vi "Calibrate Sensor Angle.vi"() -> ()   [LabVIEW 2014]
uses:
  <vilib>/Utility/AngleManip/Degrees to Radians (Scalar DBL).vi
  <vilib>/robotics/Starter Kit/2.0/9632 Host Interface/NI_Robotics_Starter Kit Host_9632_2.0.lvclass
  <vilib>/Utility/AngleManip/NI_AngleManipulation.lvlib
  <vilib>/robotics/Starter Kit/Host Interface/NI_Robotics_Starter Kit Host.lvclass
panel:
  in  "sensor motor angle":dbl(slide) caption="Sensor Motor Angle (degrees)" scale=90.0..-90.0
  in  "zero":bool
  in  "stop":bool
  # "Adjust the slider until the sensor is facing directly forward on the robot, then press Zero Angle to calibrate the sensor orientation."
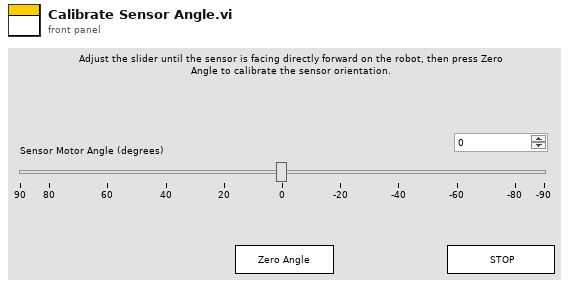
[diagram p1: front panel]
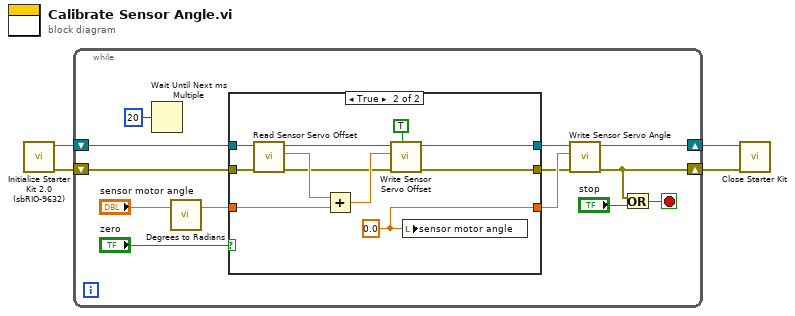
[diagram p0: block diagram]
diagram:
  n1 = call <vilib>:"Initialize Starter Kit 2.0 (sbRIO-9632).vi"() -> ("error out"=w3:errorcluster, "FPGA starter kit host 2.0 out"=w4:refnum<class "NI_Robotics_Starter Kit Host_9632_2.0.lvclass">)  [unwired: 10 in]
  n2 = while {
    shift-right: [w6] -> w2
    shift-left: w4 -> [w13]
    shift-right: [w5] -> w1
    shift-left: w3 -> [w14]
    stop <- w16 stop-if-true
    n3 = Wait Until Next ms Multiple(millisecond multiple=u32 20) -> ()  [unwired: 1 out]
    n4 = call-poly <vilib>:"Degrees to Radians.vi"("angle (deg)"="sensor motor angle") -> ("angle (rad)"=w10:dbl)  [unwired: 2 in]
    n5 = case shown="True" "zero" {
      tunnel: w14 -> [w19 w22]
      tunnel: w13 -> [w20 w23]
      tunnel: [w20 w26] -> w8
      tunnel: [w19 w24] -> w7
      tunnel: w10 -> [w18 w30]
      tunnel: [w18 w31] -> w9
      frame False {
      }
      frame True {
        w31 = 0.0 ("sensor motor angle")
        n6 = call <vilib>:"Read Sensor Servo Offset.vi"("error in (no error)"=w22, "starter kit host in"=w23) -> ("error out"=w21:errorcluster, "ccw offset angle (rad)"=w29:dbl, "starter kit host out"=w27:refnum<class "NI_Robotics_Starter Kit Host_9632_2.0.lvclass">)  [unwired: 7 in]
        n7 = Add(x=w29, y=w30) -> (x+y=w28:dbl)
        n8 = call <vilib>:"Write Sensor Servo Offset.vi"("save to file (F)"=TRUE, "error in (no error)"=w21, "ccw offset angle (rad)"=w28, "starter kit host in"=w27) -> ("error out"=w24:errorcluster, "starter kit host out"=w26:refnum<class "NI_Robotics_Starter Kit Host_9632_2.0.lvclass">)  [unwired: 6 in]
        n9 = local write "sensor motor angle"(w31) -> ()
      }
    }
    n10 = call <vilib>:"Write Sensor Servo Angle.vi"("error in (no error)"=w7, "ccw servo angle (rad)"=w9, "starter kit host in"=w8) -> ("error out"=w5:errorcluster, "starter kit host out"=w6:refnum<class "NI_Robotics_Starter Kit Host_9632_2.0.lvclass">)  [unwired: 7 in]
    n11 = Or(x=w5, y="stop") -> (x .or. y?=w16:bool)
  }
  n12 = call-dynamic "Close Starter Kit.vi"("error in (no error)"=w1, "starter kit host in"=w2) -> ()  [unwired: 9 in, 1 out]
